vi "Add single row.vi"(8 "error in (no error)":errorcluster, 10 "Row":string[](array[string]), 11 "MulColLBTable.lvclass":refnum<class "MulColLBTable.lvclass">) -> (0 "error out":errorcluster, 3 "MulColLBTable.lvclass 2":refnum<class "MulColLBTable.lvclass">)   [LabVIEW 2020, in "MulColLBTable.lvclass"]
uses:
  MulColLBTable.lvclass
  MulColLBTable.lvclass/MulColLBTable.ctl
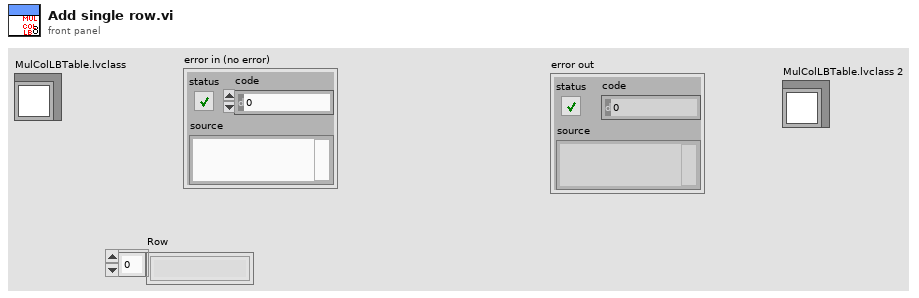
[diagram p1: front panel]
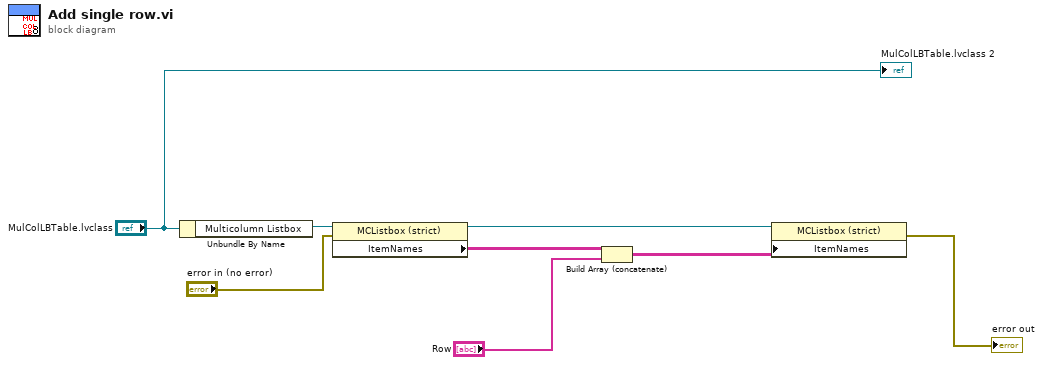
[diagram p0: block diagram]
diagram:
  n1 = Unbundle By Name("MulColLBTable.lvclass") -> ("Multicolumn Listbox"=w7:refnum<vi>)
  n2 = property class="MCListbox (strict)"(reference=w7, error in="error in (no error)") -> (reference out=w6:refnum<vi>, "ItemNames"=w5:string[][])  [unwired: 1 out]
  n3 = Build Array (concatenate)(w5, "Row") -> (w4:string[][])
  n4 = property class="MCListbox (strict)"(reference=w6, "ItemNames"=w4) -> (error out=→"error out":errorcluster)  [unwired: 1 in, 1 out]
  "MulColLBTable.lvclass 2" <- "MulColLBTable.lvclass"
